vi "ConvertToWriteByte.vi"(11 "Input":u8) -> (3 "Output":u16)   [LabVIEW 2016, in "FPGAMockGyro.lvlib"]
uses:
  FPGAMockGyro.lvlib
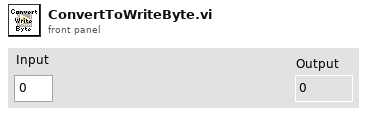
[diagram p1: front panel]
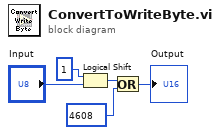
[diagram p0: block diagram]
diagram:
  n1 = Logical Shift(y=i16 1, x="Input") -> (x << y=w4:u8)
  n2 = Or(x=w4, y=u16 4608) -> (x .or. y?=→"Output":u16)
